vi "测试类型3can应答.vi"(7 "输出切换ID":u8, 8 "输入切换ID":u8) -> (3 "成功？":bool)   [LabVIEW 2010]
uses:
  全局量/全局_配置.vi
panel:
  out "开始时间":dbl format="%#.0f"
  in  "匹配CANID":u32 format="%x"
  out "接收数据":u8[](array[numeric])
  out "超时?":bool
  in  "Baudrate":u32(ring)=1000 caption="K" items=["10"=10, "20"=20, "50"=50, "100"=100, "125"=125, "250"=250, "500"=500, "800"=800, "250"=1000]
  in  "CANPort":u16
  in  "ReadTimeOut":u32=3000 caption="ms"
  in  "Synchronization":i32(ring)=1 items=["Synchronization"=1, "Asynchronization"=0]
  out "Error out":errorcluster {"code" format="%.0x"}
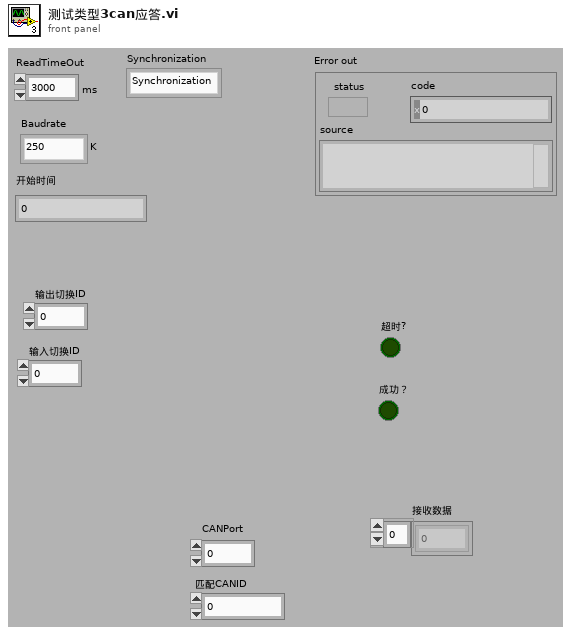
[diagram p1: front panel]
types:
  T1 = cluster{"Internal":u32, "InternalHigh":u32, "Offset":u32, "OffsetHigh":u32, "hEvent":u32}
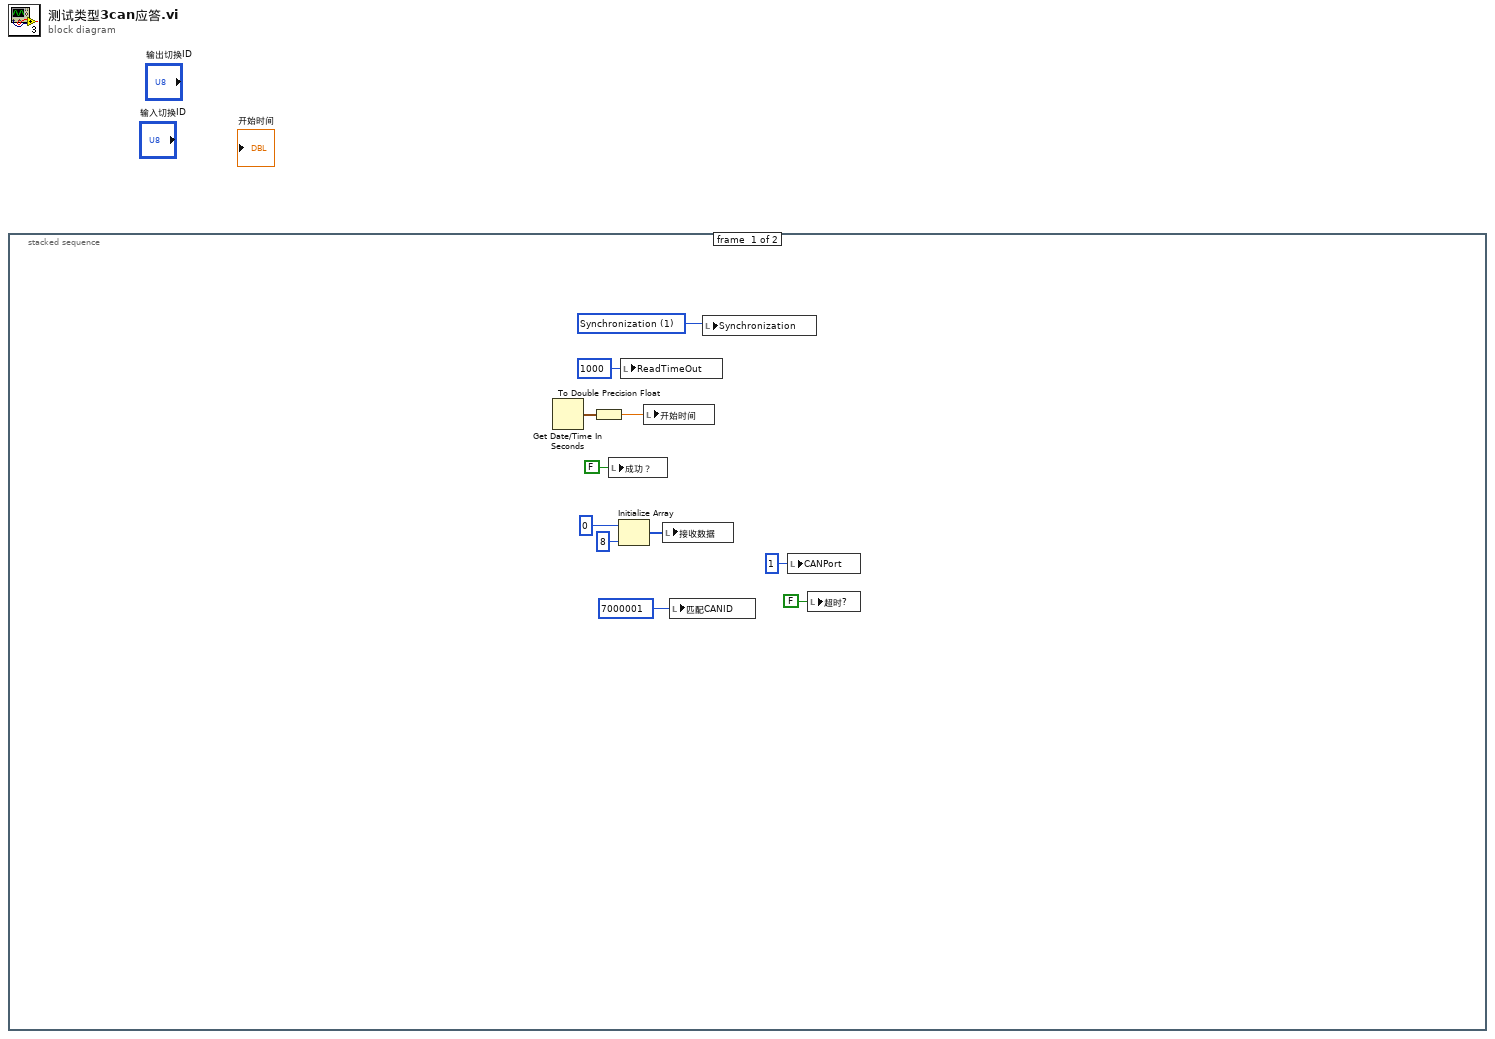
[diagram p0: block diagram]
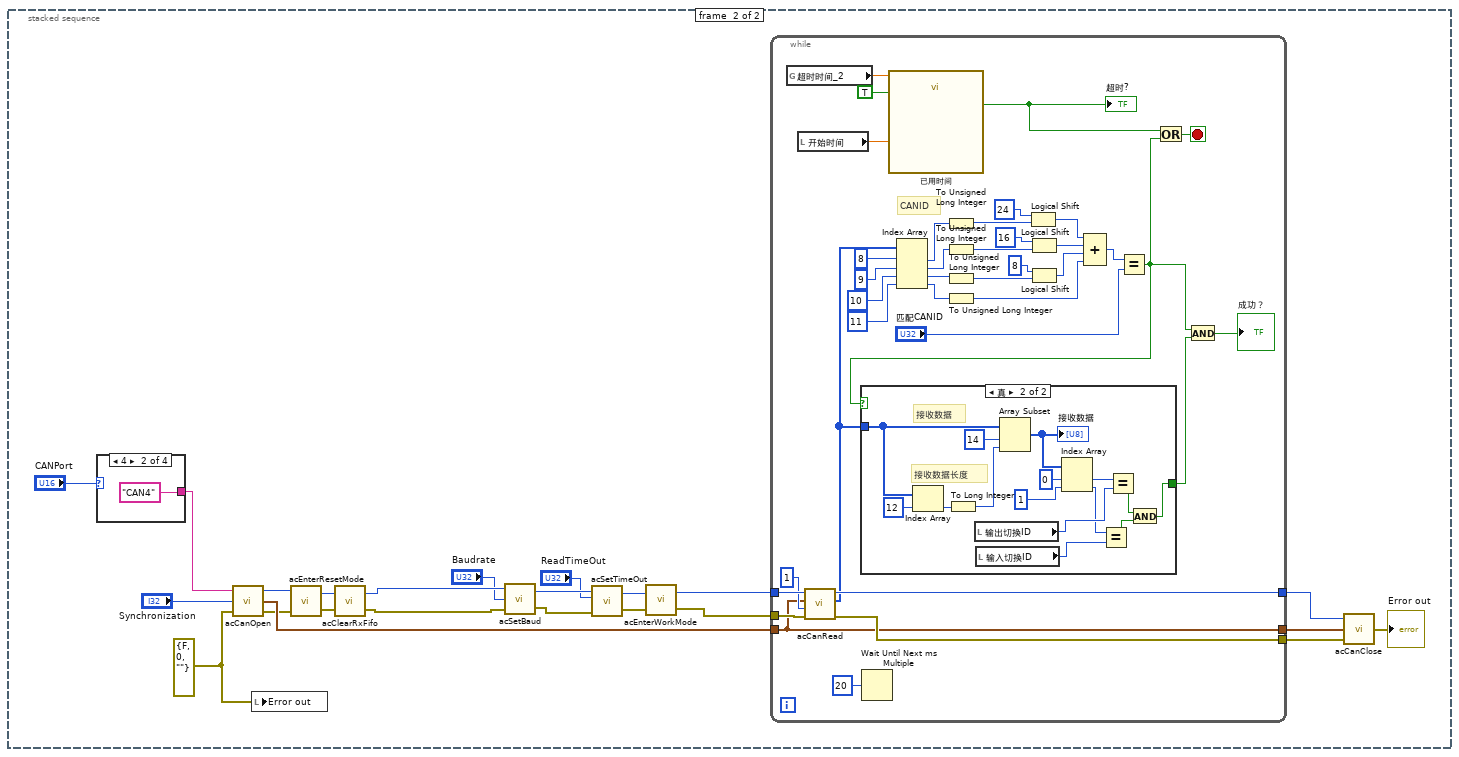
[diagram p2: hidden frame]
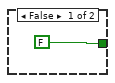
[diagram p3: hidden frame]
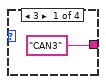
[diagram p4: hidden frame]
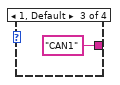
[diagram p5: hidden frame]
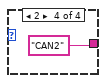
[diagram p6: hidden frame]
diagram:
  n1 = stacked-sequence {
    frame #0 {
      w3 = 1 items=["Synchronization"=1, "Asynchronization"=0] ("Synchronization")
      n2 = Get Date/Time In Seconds() -> (seconds since 1Jan1904=w7:timestamp)
      n3 = To Double Precision Float(number=w7) -> (double precision float=w8:dbl)
      n4 = local write "成功？"(FALSE ("成功？")) -> ()
      n5 = Initialize Array(u8 0, 8 ("维数大小")) -> (w6:u8[])
      n6 = local write "ReadTimeOut"(u32 1000 ("ReadTimeOut")) -> ()
      n7 = local write "开始时间"(w8) -> ()
      n8 = local write "接收数据"(w6) -> ()
      n9 = local write "匹配CANID"(7000001 ("维数大小")) -> ()
      n10 = local write "Synchronization"(w3) -> ()
      n11 = local write "CANPort"(u16 1 ("CANPort")) -> ()
      n12 = local write "超时?"(FALSE ("超时?")) -> ()
    }
    frame #1 {
      w28 = errorcluster {"status"=FALSE, "code"=0, "source"=""} ("Error in")
      n13 = case shown="4" "CANPort" {
        tunnel: ["CAN3" "CAN4" "CAN1" "CAN2"] -> w13
        frame 3 {
        }
        frame 4 {
        }
        frame 1, Default {
        }
        frame 2 {
        }
      }
      n14 = call "acCanOpen.vi"("Error in"=w28, "Synchronization"="Synchronization", "CANPort"=w13) -> ("Error out"=w29:errorcluster, "Overlapped"=w32:T1, "Handle"=w30:u32)
      n15 = local write "Error out"(w28) -> ()
      n16 = call "acEnterResetMode.vi"("Error in"=w29, "Handle  in"=w30) -> ("Error out"=w23:errorcluster, "Handle out"=w22:u32)
      n17 = call "acClearRxFifo.vi"("Error in"=w23, "Handle  in"=w22) -> ("Error out"=w20:errorcluster, "Handle out"=w21:u32)
      n18 = call "acSetBaud.vi"("Error in"=w20, "Baudrate"="Baudrate", "Handle  in"=w21) -> ("Error out"=w25:errorcluster, "Handle out"=w26:u32)
      n19 = call "acSetTimeOut.vi"("Error in"=w25, "Read TimeOut"="ReadTimeOut", "Handle  in"=w26) -> ("Error out"=w18:errorcluster, "Handle out"=w19:u32)  [unwired: 1 in]
      n20 = call "acEnterWorkMode.vi"("Error in"=w18, "Handle  in"=w19) -> ("Error out"=w16:errorcluster, "Handle out"=w17:u32)
      n21 = while {
        tunnel: [w70] -> w33
        tunnel: w32 -> [w65]
        tunnel: [w69] -> w31
        tunnel: w17 -> [w68]
        tunnel: w16 -> [w67]
        tunnel: [w65] -> w12
        stop <- w61 stop-if-true
        # "CANID"
        n22 = global read "全局_配置.vi" "超时时间_2"() -> (w63:dbl)
        n23 = local read "开始时间"() -> (w62:dbl)
        n24 = call "acCanRead.vi"("Error in"=w67, "ReadCount"=u32 1 ("接收CAN帧数 2"), "Overlapped"=w65, "Handle  in"=w68) -> ("Error out"=w69:errorcluster, "MSG"=w39:u8[], "Handle out"=w70:u32)  [unwired: 1 out]
        n25 = Wait Until Next ms Multiple(millisecond multiple=u32 20 ("毫秒倍数")) -> ()  [unwired: 1 out]
        n26 = call "已用时间"("Time Target (s)"=w63, "Reset"=TRUE, "Set Start Time (s)"=w62) -> ("Time has Elapsed"=w35:bool)  [unwired: 9 in, 7 out]
        "超时?" <- w35
        n27 = Index Array(array=w39, index #1=8 ("索引"), index #2=9 ("索引"), index #3=10 ("索引"), index #4=11 ("索引")) -> (element #1=w46:u8, element #2=w45:u8, element #3=w42:u8, element #4=w41:u8)
        n28 = To Unsigned Long Integer(number=w46) -> (unsigned 32bit integer=w47:u32)
        n29 = To Unsigned Long Integer(number=w45) -> (unsigned 32bit integer=w44:u32)
        n30 = To Unsigned Long Integer(number=w42) -> (unsigned 32bit integer=w43:u32)
        n31 = To Unsigned Long Integer(number=w41) -> (unsigned 32bit integer=w40:u32)
        n32 = Logical Shift(y=i8 24, x=w47) -> (x << y=w51:u32)
        n33 = Logical Shift(y=i8 16, x=w44) -> (x << y=w52:u32)
        n34 = Logical Shift(y=i8 8, x=w43) -> (x << y=w50:u32)
        n35 = Compound Arithmetic op=ADD(w51, w52, w50, w40) -> (w49:u32)
        n36 = Equal?(x=w49, y="匹配CANID") -> (x = y?=w38:bool)
        n37 = case shown="真" w38 {
          tunnel: w39 -> [_ w82]
          tunnel: [FALSE w72] -> w37
          frame False {
          }
          frame True {
            # "接收数据"
            # "接收数据长度"
            n38 = Index Array(array=w82, index=12 ("索引")) -> (element=w84:u8)
            n39 = To Long Integer(number=w84) -> (32bit integer=w83:i32)
            n40 = local read "输出切换ID"() -> (w77:u8)
            n41 = local read "输入切换ID"() -> (w75:u8)
            n42 = Array Subset(array=w82, index=14 ("索引"), length=w83) -> (w81:u8[])
            "接收数据" <- w81
            n43 = Index Array(array=w81, index #1=0 ("索引"), index #2=1 ("索引")) -> (element #1=w79:u8, element #2=w76:u8)
            n44 = Equal?(x=w76, y=w75) -> (x = y?=w73:bool)
            n45 = Equal?(x=w79, y=w77) -> (x = y?=w74:bool)
            n46 = And(x=w74, y=w73) -> (x .and. y?=w72:bool)
          }
        }
        n47 = Or(x=w35, y=w38) -> (x .or. y?=w61:bool)
        n48 = And(x=w38, y=w37) -> (x .and. y?=→"成功？":bool)
      }
      n49 = call "acCanClose.vi"("Error in"=w31, "Overlapped"=w12, "Handle  in"=w33) -> ("Error out"=→"Error out":errorcluster)
    }
  }
